vi "Constructor.vi"(5 "TimeZoneInfoId":string, 7 "ComparisonType":T1, 8 "error in":errorcluster, 9 "HigherBound":timestamp, 10 "LowerBound":timestamp, 11 "Name":string) -> (0 "error out":errorcluster, 3 "DateTimeMeasureLimit":refnum<class "DateTimeMeasureLimit.lvclass">)   [LabVIEW 2021, in "ProligentXMLGenerator.lvlib" / "DateTimeMeasureLimit.lvclass"]
uses:
  DateTimeMeasureLimit.lvclass
  DateTimeMeasureLimit.lvclass/DateTimeMeasureLimit.ctl
  MeasureLimit/MeasureLimit.lvclass
  Base/DateTime/DateTime.lvclass
  Data.ctl
  RangeMeasureLimit/RangeMeasureLimit.lvclass
  C:/Projects/proligent-xml-generator-labview/src/ProligentXMLGenerator/Measure/RangeMeasureLimit/RangeMeasureLimit.lvclass
  C:/Projects/proligent-xml-generator-labview/src/ProligentXMLGenerator/Measure/MeasureLimit/MeasureLimit.lvclass
  RangeMeasureLimit/ComparisonType.ctl
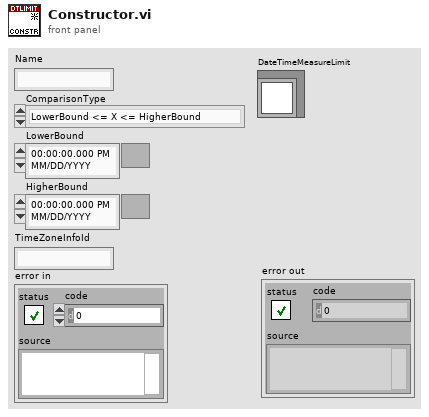
[diagram p1: front panel]
types:
  T1 = typedef "ProligentXMLGenerator.lvlib/RangeMeasureLimit.lvclass/ComparisonType.ctl" = enum16{"LowerBound <= X <= HigherBound", "LowerBound < X <= HigherBound", "LowerBound <= X < HigherBound", "LowerBound < X < HigherBound", "LowerBound <= X", "LowerBound < X", "X <= HigherBound", "X < HigherBound", "X == HigherBound", "X != HigherBound", "X <= LowerBound OR HigherBound <= X", "X < LowerBound OR HigherBound <= X", "X <= LowerBound OR HigherBound < X", "X < LowerBound OR HigherBound < X"}
  T2 = typedef "ProligentXMLGenerator.lvlib/DateTimeMeasureLimit.lvclass/Data.ctl" = cluster{"LowerBound":refnum<class "DateTime.lvclass">, "HigherBound":refnum<class "DateTime.lvclass">}
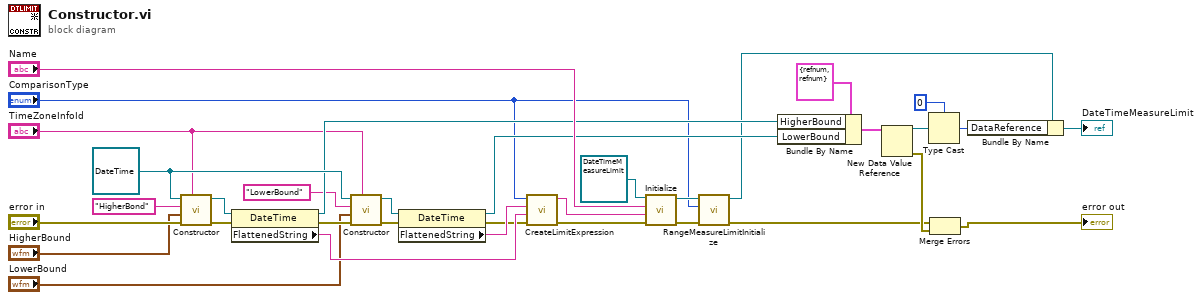
[diagram p0: block diagram]
diagram:
  w21 = refnum<class "DateTime.lvclass"> refnum ("ProligentResultProcessor:DateTime")
  n1 = call-dynamic "Constructor.vi"("TimeZoneInfoId"="TimeZoneInfoId", "error in"="error in", "Value"="HigherBound", "Name"="HigherBond", "DateTime in"=w21) -> ("error out"=w22:errorcluster, "DateTime out"=w17:refnum<class "DateTime.lvclass">)  [unwired: 5 in]
  n2 = property class="DateTime"(reference=w17, error in=w22) -> (reference out=w9:refnum<class "DateTime.lvclass">, error out=w18:errorcluster, "FlattenedString"=w16:string)
  n3 = call-dynamic "Constructor.vi"("TimeZoneInfoId"="TimeZoneInfoId", "error in"=w18, "Value"="LowerBound", "Name"="LowerBound", "DateTime in"=w21) -> ("error out"=w13:errorcluster, "DateTime out"=w14:refnum<class "DateTime.lvclass">)  [unwired: 5 in]
  n4 = property class="DateTime"(reference=w14, error in=w13) -> (reference out=w10:refnum<class "DateTime.lvclass">, error out=w11:errorcluster, "FlattenedString"=w12:string)
  n5 = call "CreateLimitExpression.vi"("error in"=w11, "HigherBound"=w16, "LowerBound"=w12, "ComparisonType"="ComparisonType") -> ("error out"=w26:errorcluster, "LimitExpression"=w25:string)  [unwired: 6 in]
  n6 = call "Initialize.vi"("error in"=w26, "LimitExpression"=w25, "Name"="Name", "MeasureLimit in"=refnum<class "DateTimeMeasureLimit.lvclass"> refnum ("ProligentResultProcessor:DateTimeMeasureLimit")) -> ("error out"=w4:errorcluster, "MeasureLimit out"=w24:refnum<class "DateTimeMeasureLimit.lvclass">)  [unwired: 6 in]
  n7 = call "RangeMeasureLimitInitialize.vi"("error in"=w4, "ComparisonType"="ComparisonType", "RangeMeasureLimit in"=w24) -> ("error out"=w3:errorcluster, "RangeMeasureLimit out"=w5:refnum<class "DateTimeMeasureLimit.lvclass">)  [unwired: 7 in]
  n8 = Bundle By Name(cluster=T2 {"LowerBound"=refnum, "HigherBound"=refnum} ("Data"), "HigherBound"=w9, "LowerBound"=w10) -> (w30:T2)
  n9 = New Data Value Reference(data value=w30) -> (data value reference=w31:refnum<data-value>, error out=w34:errorcluster)  [unwired: 1 in]
  n10 = Type Cast(type=u64 0, x=w31) -> (*(type *) &x=w33:u64)
  n11 = Merge Errors(w3, w34) -> (→"error out":errorcluster)
  n12 = Bundle By Name(cluster=w5, "DataReference"=w33) -> (→"DateTimeMeasureLimit":refnum<class "DateTimeMeasureLimit.lvclass">)
